vi "Script Get Module Timeout Value.vi"(8 "error in":errorcluster, 10 "vi path":path, 11 "application reference (local)":refnum<vi>) -> (0 "error out":errorcluster, 3 "Module Timeout":i32)   [LabVIEW 2019, in "Panther Dashboard.lvlib"]
uses:
  Panther Dashboard.lvlib
  <vilib>/Utility/traverseref.llb/TRef TravTarget.ctl
  <vilib>/Utility/traverseref.llb/VI Scripting - Traverse.lvlib
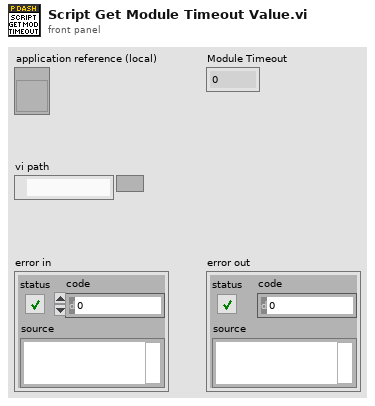
[diagram p1: front panel]
types:
  T1 = typedef "TRef TravTarget.ctl" = enum16{"FP", "BD", "Other"}
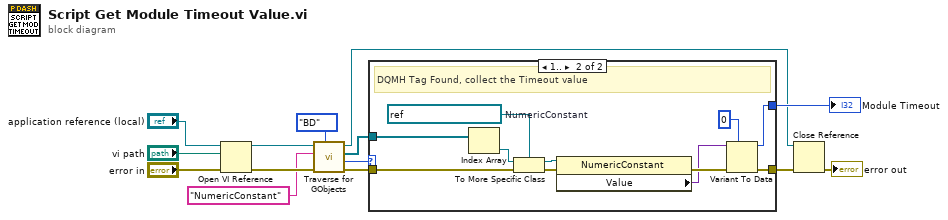
[diagram p0: block diagram]
diagram:
  n1 = Open VI Reference(application reference (local)="application reference (local)", vi path="vi path", error in (no error)="error in") -> (vi reference=w4:refnum<vi>, error out=w11:errorcluster)  [unwired: 3 in]
  n2 = call <vilib>:"Traverse for GObjects.vi"("Traverse Target"=TRef_TravTarget."BD", "error in (no error)"=w11, "Class Name"="NumericConstant", "VI Refnum"=w4) -> ("error out"=w14:errorcluster, "# of Refs"=w8:i32, "References"=w7:refnum<vi>[], "dup VI Refnum"=w1:refnum<vi>)  [unwired: 4 in]
  n3 = case shown="1.." w8 {
    tunnel: w14 -> [w15 w26]
    tunnel: w7 -> [_ w20]
    tunnel: [w15 w23] -> w13
    tunnel: [_ w16] -> w9
    frame Default {
    }
    frame 1.. {
      w22 = refnum<vi> refnum  # NumericConstant
      # "DQMH Tag Found, collect the Timeout value"
      n4 = Index Array(array=w20) -> (element=w19:refnum<vi>)  [unwired: 1 in]
      n5 = To More Specific Class(target class=w22, reference=w19, error in=w26) -> (specific class reference=w21:refnum<vi>, error out=w25:errorcluster)
      n6 = property class="NumericConstant"(reference=w21, error in=w25) -> (error out=w24:errorcluster, "Value"=w18:variant)  [unwired: 1 out]
      n7 = Variant To Data(error in=w24, type=0, Variant=w18) -> (data=w16:i32, error out=w23:errorcluster)
    }
  }
  "Module Timeout" <- w9
  n8 = Close Reference(reference=w1, error in (no error)=w13) -> (error out=→"error out":errorcluster)
